vi "PH_Sound.PlayTone.vi"(0 "VI in":refnum<vi>, 2 "tone":T1=261.6 items=["c"=130.8, "cis"=138.6, "d"=146.8, "es"=155.6, "e"=164.8, "f"=174.6, "fis"=185.0, "g"=196.0, "as"=207.6, "a"=220.0, "b"=233.1, "h"=246.9, "c'"=261.6, "cis'"=277.2, "d'"=293.7, "es'"=311.1, "e'"=329.6, "f'"=349.2, "fis'"=370.0, "g'"=392.0, "as'"=415.3, "a'"=440.0, "b'"=466.2, "h'"=493.9, "c''"=523.3, "cis''"=554.4, "d''"=587.3, "es''"=622.3, "e''"=659.3, "f''"=689.5, "fis''"=740.0, "g''"=784.0, "as''"=830.6, "a''"=880.0, "b''"=932.3, "h''"=987.8, "c'''"=1047.0], 4 "length [ms]":i32=200, 5 "error in":errorcluster) -> (14 "VI out":refnum<vi>, 19 "error out":errorcluster)   [LabVIEW 2014, in "PH_Sound.lvlib"]
doc: "This VI plays a tone (frequency) of several length with a settable amplitude"
uses:
  PH_Sound.lvlib
  PH_Sound.3Oktaves.ctl
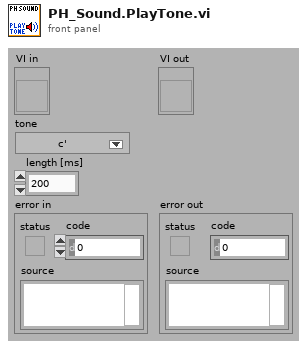
[diagram p1: front panel]
types:
  T1 = typedef "PH_Sound.lvlib/PH_Sound.3Oktaves.ctl" = dbl
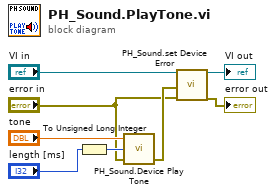
[diagram p0: block diagram]
diagram:
  n1 = To Unsigned Long Integer(number="length [ms]") -> (unsigned 32bit integer=w4:u32)
  n2 = call "PH_Sound.Device Play Tone.vi"("error in"="error in", "Length [ms]"=w4, "tone"="tone") -> ("Device error out"=w6:errorcluster)  [unwired: 2 in]
  n3 = call "PH_Sound.set Device Error.vi"("VI in"="VI in", "Device error"=w6, "error in"="error in") -> ("VI out"=→"VI out":refnum<vi>, "error out"=→"error out":errorcluster)  [unwired: 15 in]
